vi "aad.vi"() -> ()   [LabVIEW 2024]
panel:
  out "return count":u32
  out "Data string":string
  in  "baud rate (9600)":u32=19200
  in  "VISA resource name":refnum<visa-resource-name>="VirtualDevice1"
  in  "Start/Stop":bool caption="Boolean 3"
  out "LEDs":bool[](array[boolean])
  in  "Numeric":i32 caption="ASCII code"
  in  "Gauge":dbl(knob) caption="Delay\nDelay" scale=0.0..1.0
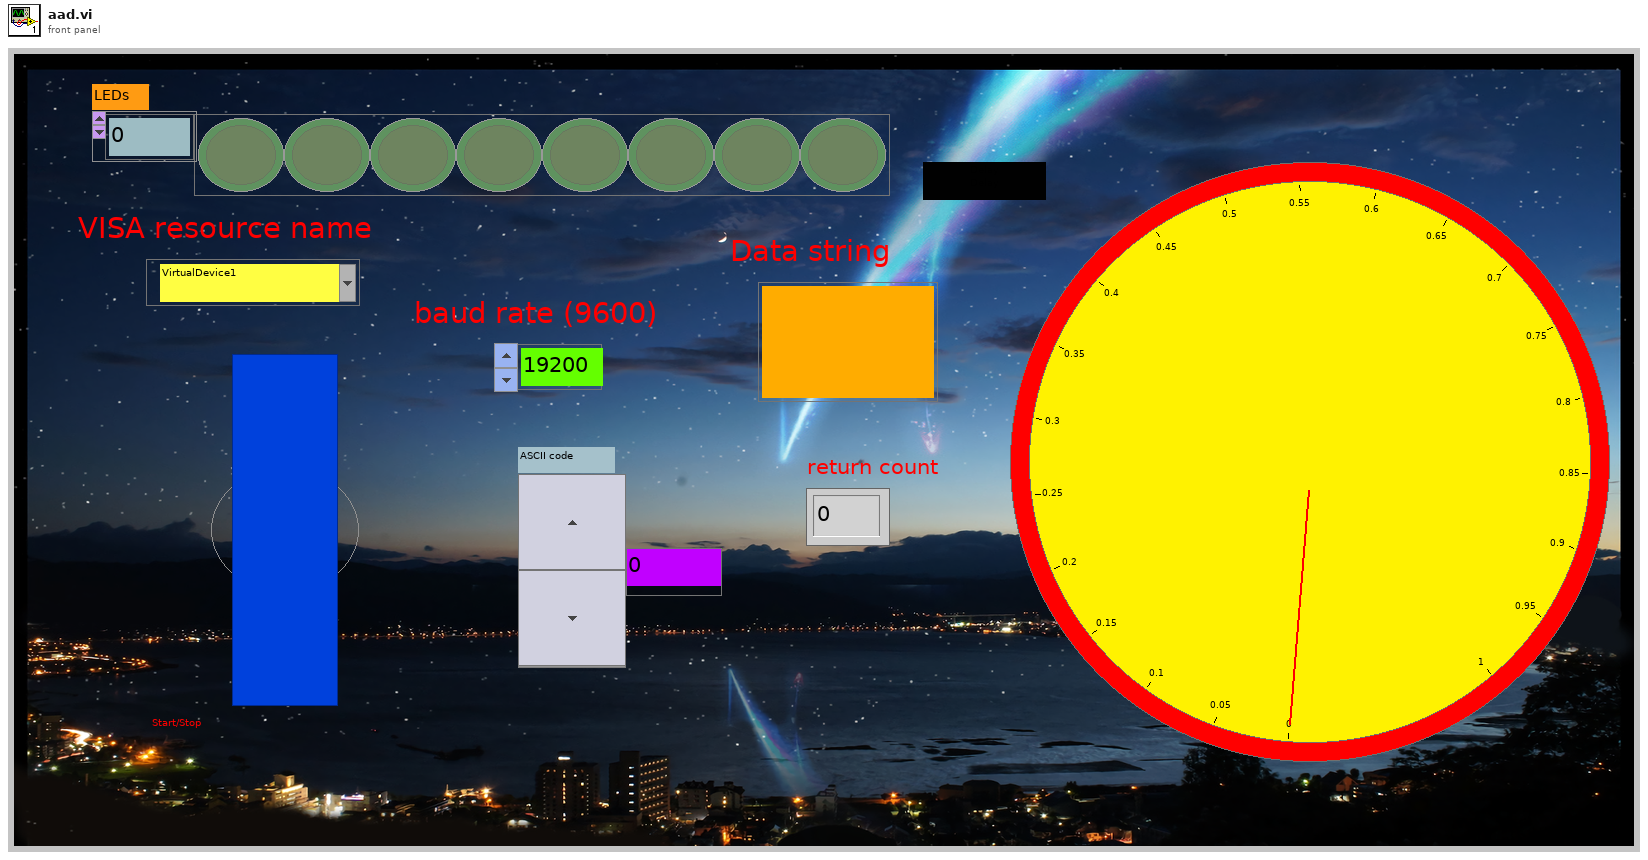
[diagram p1: front panel]
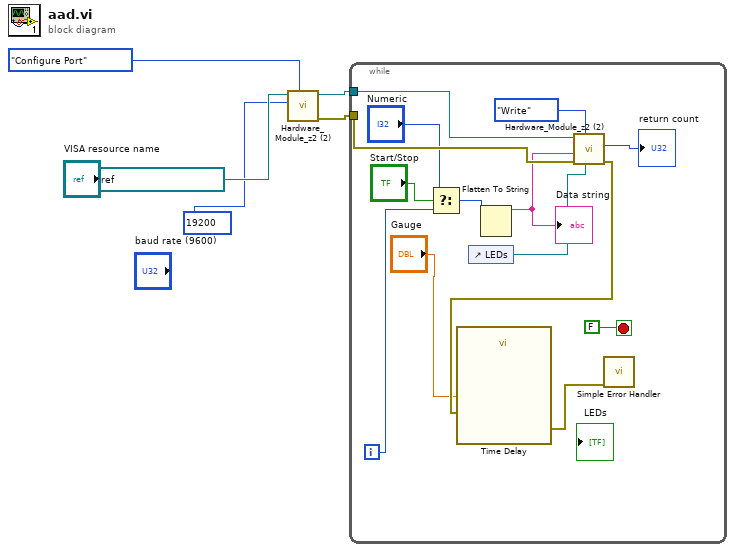
[diagram p0: block diagram]
diagram:
  n1 = call "Hardware_Module_z2 (2).vi"("State"=enum16{"Configure Port", "Write", "Close"}."Configure Port", "baud rate (9600)"=u32 19200, "VISA resource name"=refnum<visa-resource-name> "VirtualDevice1") -> ("error out"=w3:errorcluster, "VISA resource name out"=w2:refnum<visa-resource-name>)  [unwired: 6 in, 1 out]
  n2 = while {
    tunnel: w3 -> [w18]
    tunnel: w2 -> [w17]
    i -> [w11]
    stop <- FALSE stop-if-true
    n3 = Select(t="Numeric", s="Start/Stop", f=w11) -> (s? t:f=w13:i32)
    n4 = control-ref of="LEDs"() -> (w9:refnum<vi>)
    n5 = Flatten To String(anything=w13) -> (data string=w8:string)  [unwired: 3 in, 2 out]
    "Data string" <- w8
    n6 = call "Hardware_Module_z2 (2).vi"("LEDs"=w9, "State"=enum16{"Configure Port", "Write", "Close"}."Write", "error in (no error)"=w18, "write buffer"=w8, "VISA resource name"=w17) -> ("error out"=w16:errorcluster, "return count"=→"return count":u32)  [unwired: 4 in, 1 out]
    n7 = call "Time Delay"("error in (no error)"=w16, "Delay Time (s)"="Gauge") -> ("error out"=w6:errorcluster)  [unwired: 9 in]
    n8 = call <vilib>:"Simple Error Handler.vi"("error in (no error)"=w6) -> ()  [unwired: 4 in, 5 out]
  }
